vi "detector_get_data_dimensions.vi"(8 "error in (no error)":errorcluster, 11 "hydraharp in":refnum<class "hydraharp.lvclass">) -> (0 "error out":errorcluster, 1 "data_type":T1, 2 "dims":u32[](array[numeric]), 3 "hydraharp out":refnum<class "hydraharp.lvclass">)   [LabVIEW 2015, in "hydraharp.lvclass"]
uses:
  hydraharp.lvclass
  detector/data_types_tdef.ctl
  hydraharp.lvclass/hydraharp.ctl
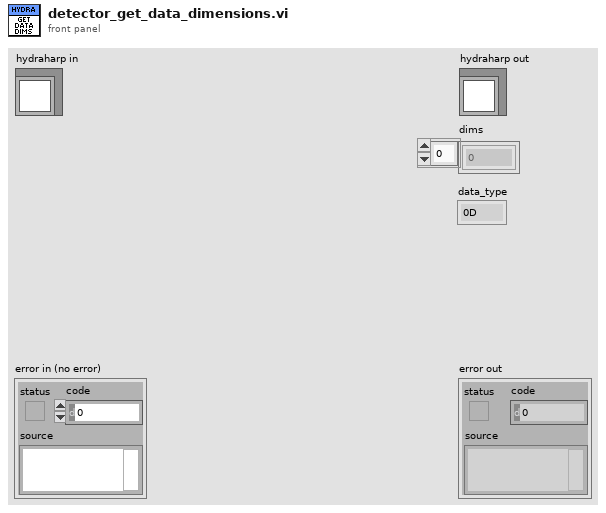
[diagram p1: front panel]
types:
  T1 = typedef "data_types_tdef.ctl" = enum16{"0D", "1D", "2D"}
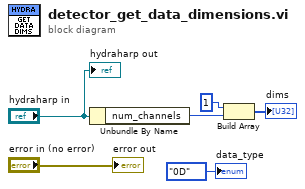
[diagram p0: block diagram]
diagram:
  n1 = Unbundle By Name("hydraharp in") -> ("num_channels"=w4:i32)
  n2 = Build Array(u32 1 ("element"), w4) -> (→"dims":u32[])
  "error out" <- "error in (no error)"
  "hydraharp out" <- "hydraharp in"
  "data_type" <- data_types_tdef."0D" ("data_type")
